vi "SPT-Create Pulse.vi"(0 "SPT.Properties":T1, 7 "Fs (Hz)":dbl, 11 "error in (no error)":errorcluster) -> (8 "Pulse":dbl[](array[numeric]), 15 "error out":errorcluster)   [LabVIEW 2015]
uses:
  SPT-Properties.ctl
  SPT-Shape.ctl
  Utility VIs/Math VIs/LinSpace (x0-dx-npts).vi
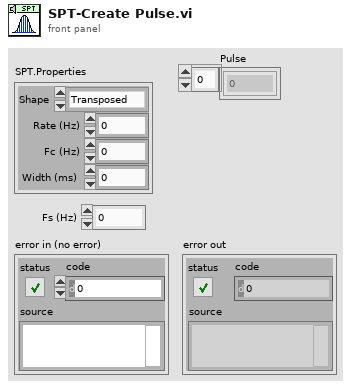
[diagram p1: front panel]
types:
  T1 = typedef "SPT-Properties.ctl" = cluster{"Shape":T2, "Rate (Hz)":dbl, "Fc (Hz)":dbl, "Width (ms)":dbl}
  T2 = typedef "SPT-Shape.ctl" = enum16{"Transposed", "Alpha", "Gabor"}
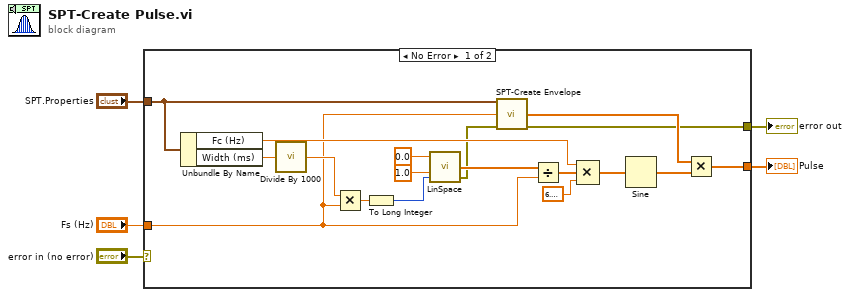
[diagram p0: block diagram]
diagram:
  n1 = case shown="No Error" "error in (no error)" {
    selector: "error in (no error)" -> [_ w24]
    tunnel: "SPT.Properties" -> [w13 _]
    tunnel: "Fs (Hz)" -> [w6 _]
    tunnel: [w7 w24] -> w2
    tunnel: [w9 _] -> w1
    frame No Error {
      n2 = Unbundle By Name(w13) -> ("Fc (Hz)"=w14:dbl, "Width (ms)"=w23:dbl)
      n3 = call "Divide By 1000.vi"("X"=w23) -> ("X/1000"=w17:dbl)
      n4 = Multiply(x=w17, y=w6) -> (x*y=w22:dbl)
      n5 = To Long Integer(number=w22) -> (32bit integer=w18:i32)
      n6 = call-poly "LinSpace.vi"("npts"=w18, "dx"=1.0, "x0"=0.0) -> ("error out"=w8:errorcluster, "Array"=w19:dbl[])  [unwired: 1 in]
      n7 = call "SPT-Create Envelope.vi"("SPT.Properties"=w13, "Fs (Hz)"=w6, "error in (no error)"=w8) -> ("Env"=w10:dbl[], "error out"=w7:errorcluster)  [unwired: 11 in]
      n8 = Divide(x=w19, y=w6) -> (x/y=w16:dbl[])
      n9 = Compound Arithmetic op=MULTIPLY(w14, w16, 6.283185307179586) -> (w12:dbl[])
      n10 = Sine(x=w12) -> (sin(x)=w11:dbl[])
      n11 = Multiply(x=w10, y=w11) -> (x*y=w9:dbl[])
    }
    frame Error {
    }
  }
  "error out" <- w2
  "Pulse" <- w1
